vi "Secondary Joystick Control.vi"(8 "Bottom Limit":bool, 9 "Top limit":bool, 10 "Reset Encoder?":bool, 11 "Top Stop":bool) -> ()   [LabVIEW 2013]
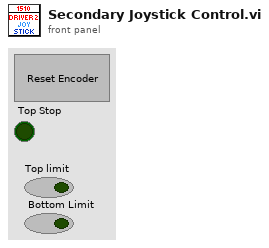
[diagram p1: front panel]
types:
  T1 = typedef "WPI_JoystickButtonState.ctl" = cluster{"Button 1":bool, "Button 2":bool, "Button 3":bool, "Button 4":bool, "Button 5":bool, "Button 6":bool, "Button 7":bool, "Button 8":bool, "Button 9":bool, "Button 10":bool, "Button 11":bool, "Button 12":bool}
  T2 = cluster{"Axes":cluster{"X Axis":dbl, "Y Axis":dbl, "Throttle":dbl, "Unused":dbl, "Unused":dbl, "Unused":dbl}, "Buttons":T1}
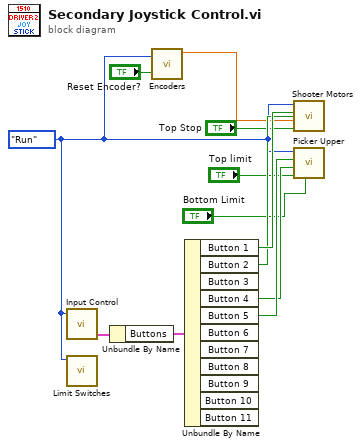
[diagram p0: block diagram]
diagram:
  w6 = enum16{"Open", "Run", "End"}."Run" ("State")
  n1 = call "Input Control.vi"("State"=w6) -> ("Secondary Joystick"=w12:T2)  [unwired: 2 in, 2 out]
  n2 = call "Limit Switches.vi"("State Control"=w6) -> ()  [unwired: 7 in, 4 out]
  n3 = Unbundle By Name(w12) -> ("Buttons"=w11:T1)
  n4 = call "Encoders.vi"("State Control"=w6, "Reset Encoder?"="Reset Encoder?") -> ("Encoder Degrees"=w5:dbl)  [unwired: 3 out]
  n5 = Unbundle By Name(w11) -> ("Button 1"=w10:bool, "Button 2"=w9:bool, "Button 4"=w7:bool, "Button 5"=w8:bool)  [unwired: 7 out]
  n6 = call "Shooter Motors.vi"("State Control"=w6, "Fire"=w10, "Return"=w5, "Top Stop"="Top Stop", "Encoder"=w9) -> ()  [unwired: 2 out]
  n7 = call "Picker Upper.vi"("Battom Limit"="Bottom Limit", "Top limit"="Top limit", "Down"=w7, "Up"=w8, "State Control"=w6) -> ()  [unwired: 7 in]
